vi "MensagemVitoriaOuEmpate.vi"(9 "Nome do Jogador":string, 11 "Selecao":string) -> ()   [LabVIEW 2011]
doc: "VI que mostra as mensagem de vitória, derrota ou empate."
panel:
  in  "OK":bool
  in  "Tab":enum32{"Venceu", "Empate", "ComputadorVenceu"}(tab)
  out "Mensagem":string
  # "Deu Velha"
  # "Que pena, você perdeu."
  # "Tente novamente."
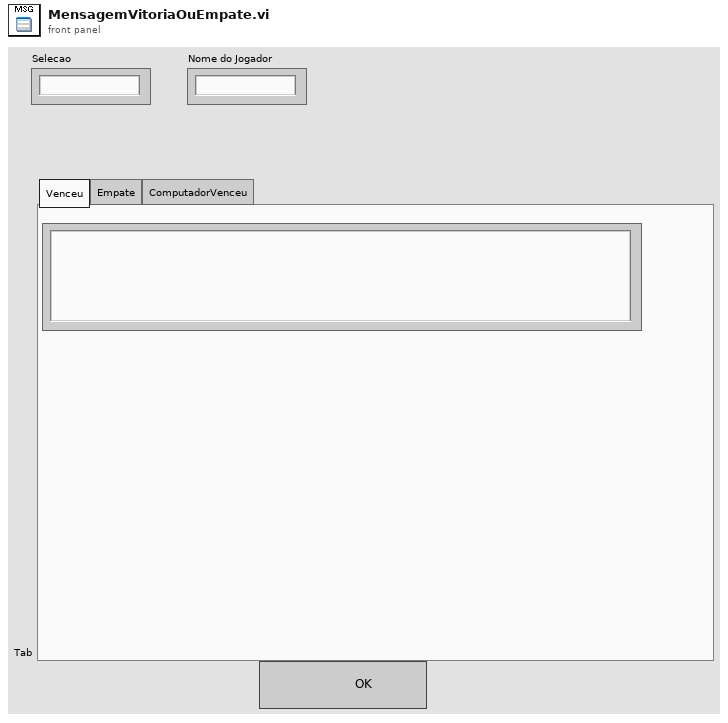
[diagram p1: front panel]
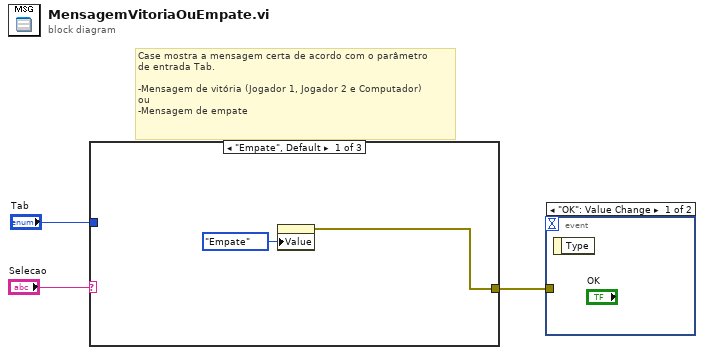
[diagram p0: block diagram]
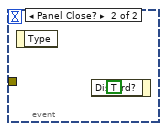
[diagram p2: hidden frame]
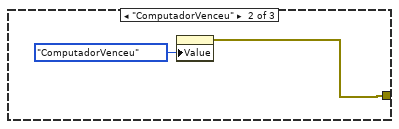
[diagram p3: hidden frame]
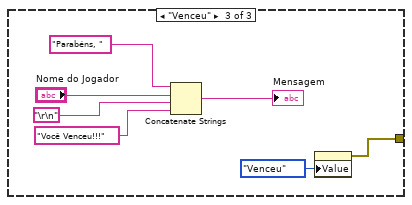
[diagram p4: hidden frame]
diagram:
  # "Case mostra a mensagem certa de acordo com o parâmetro\nde entrada Tab.\n\n-Mensagem de vitória (Jogador 1, Jogador 2 e Computador)\nou \n-Mensagem de empate"
  n1 = case shown="\"Empate\", Default" "Selecao" {
    tunnel: "Tab" -> [_ _ _]
    tunnel: [w5 w6 w10] -> w1
    frame "Empate", Default {
      n2 = property on="Tab" class="TabCtl (strict)"("Value"=enum32{"Venceu", "Empate", "ComputadorVenceu"}."Empate") -> (error out=w5:errorcluster)  [unwired: 2 in, 1 out]
    }
    frame "ComputadorVenceu" {
      n3 = property on="Tab" class="TabCtl (strict)"("Value"=enum32{"Venceu", "Empate", "ComputadorVenceu"}."ComputadorVenceu") -> (error out=w6:errorcluster)  [unwired: 2 in, 1 out]
    }
    frame "Venceu" {
      n4 = Concatenate Strings("Parabéns, " ("string"), "Nome do Jogador", "\r\n", "Você Venceu!!!" ("string")) -> (→"Mensagem":string)
      n5 = property on="Tab" class="TabCtl (strict)"("Value"=enum32{"Venceu", "Empate", "ComputadorVenceu"}."Venceu") -> (error out=w10:errorcluster)  [unwired: 2 in, 1 out]
    }
  }
  n6 = event shown="[0] \"OK\": Value Change" {
    selector: _ -> [_ _]
    dyn-events: _ -> [_ _]
    timeout: _ -> [_ _]
    tunnel: w1 -> [_ _]
    event "OK": Value Change {
      n7 = event-data() -> ()  [unwired: 1 in, 1 out]
    }
    event Panel Close? {
      n8 = event-data() -> ()  [unwired: 1 in, 1 out]
      n9 = event-data("Discard?"=TRUE) -> ()  [unwired: 1 in, 1 out]
    }
  }
